vi "Test_LocalPathMapping.vi"(8 "error in (no error)":errorcluster) -> (0 "error out":errorcluster)   [LabVIEW 2013]
uses:
  <vilib>/addons/_JKI Toolkits/Caraya/classes/Assert/Assert Equal Value_Variant.vi
  <vilib>/addons/_JKI Toolkits/Caraya/classes/Test/Test.lvclass
  <vilib>/addons/_JKI Toolkits/Caraya/classes/Assert/Assert.lvclass
  source/uri/URI.lvclass
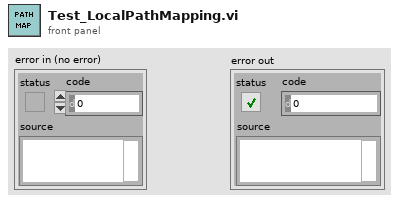
[diagram p1: front panel]
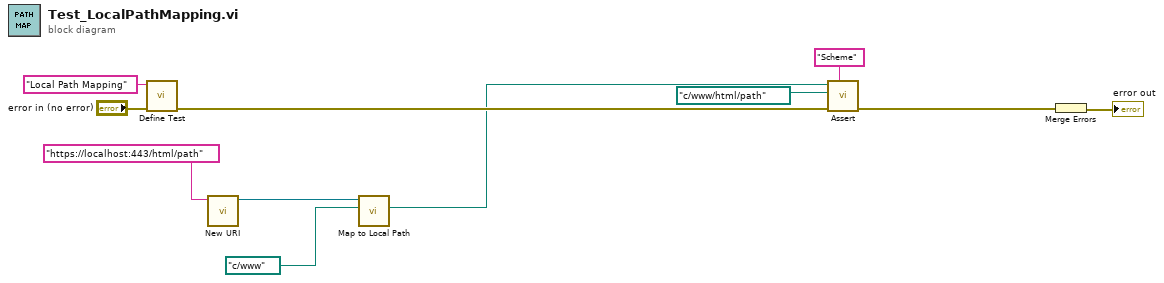
[diagram p0: block diagram]
diagram:
  n1 = call <vilib>:"Define Test.vi"("error in (no error)"="error in (no error)", "Label (VI Title)"="Local Path Mapping") -> ("error out"=w6:errorcluster)  [unwired: 9 in]
  n2 = call "New URI.vi"("URI"="https://localhost:443/html/path") -> ("URI"=w4:refnum<class "URI.lvclass">)  [unwired: 9 in, 1 out]
  n3 = call "Map to Local Path.vi"("Local Path"=path "c:/www", "URI in"=w4) -> ("Mapped Local Path"=w2:path)  [unwired: 6 in, 3 out]
  n4 = call-poly <vilib>:"Assert.vi"("Label"="Scheme" ("URI"), "error in (no error)"=w6, "Y"=path "c:/www/html/path", "X"=w2) -> ("error out"=w7:errorcluster)  [unwired: 7 in]
  n5 = Merge Errors(w7) -> (→"error out":errorcluster)
